vi "N4_X01.vi"(4 "error in":T15, 7 "Command":T16) -> (0 "error out":T15, 3 "Response":T13)   [LabVIEW 2018]
uses:
  MOKO_LabViewLibrary/MokoLowLevel/MokoLowLovelControl/MLLC_Command.ctl
  MOKO_LabViewLibrary/MokoLowLevel/MokoLowLovelControl/MLLC_Error.ctl
  MOKO_LabViewLibrary/MokoLowLevel/MokoLowLovelControl/MLLC_Mode.ctl
  MOKO_LabViewLibrary/MokoLowLevel/MokoLowLovelControl/MLLC_Response.ctl
  MOKO_LabViewLibrary/MokoLowLevel/MokoLowLovelControl/MLLC_DriverName.ctl
  MOKO_LabViewLibrary/MokoLowLevel/MokoLowLovelControl/MLLC_Request.ctl
  MOKO_LabViewLibrary/MokoLowLevel/MokoLowLovelControl/MLLC_ErrorCode.ctl
  MOKO_LabViewLibrary/MokoLowLevel/MokoLowLovelControl/MLLC_ResponseInit.ctl
  MOKO_LabViewLibrary/MokoLowLevel/MokoLowLovelControl/MLLC_ConnectCluster.ctl
  MOKO_LabViewLibrary/MokoLowLevel/MokoLowLovelControl/MLLC_InterfaceType.ctl
  MOKO_LabViewLibrary/MokoLowLevel/MokoLowLovelControl/MLLC_OpenedSession.ctl
  MOKO_LabViewLibrary/MokoLowLevel/MokoLowLovelControl/MLLC_InterfaceSettings.ctl
  MOKO_LabViewLibrary/MokoLowLevel/MokoLowLovelControl/MLLC_InterfaceKind.ctl
  MOKO_LabViewLibrary/MokoLowLevel/MokoLowLovelControl/MLLC_Boolean.ctl
  MOKO_LabViewLibrary/MokoLowLevel/MokoLowLovelControl/MLLC_Delay.ctl
panel:
  in  "Settings":T8={"Saved Data"=variant, "Permanent data"={"Connect"={"InterfaceType"=enum."VISA", "OpenedSession"="COM1", "InterfaceSettings"={"Interface"=enum."RS232", "EOS 4 read"=enum."LF (\\n)", "EOS 4 write"=enum."LF (\\n)", "TMO, ms"=10000, "Sett"=variant(cluster{"Baud Rate":u32, "Data Bits":u16, "Parity":u16, "Stop Bits":u16, "Flow Control":u16, "Eho":bool} {"Baud Rate"=75, "Data Bits"=0, "Parity"=0, "Stop Bits"=0, "Flow Control"=0, "Eho"=FALSE})}}, "RangeAuto"=TRUE, "SwitchOFF"=TRUE, "Range"=0.0}}
  in  "ResponseInit":T9="N4-101"
  in  "Error Code":T10=5470
  in  "Request":T11="IDN?"
  in  "Driver Name":T12="N4_101"
  in  "Mode":T14=enum."Check"
  # "Í4-X01"
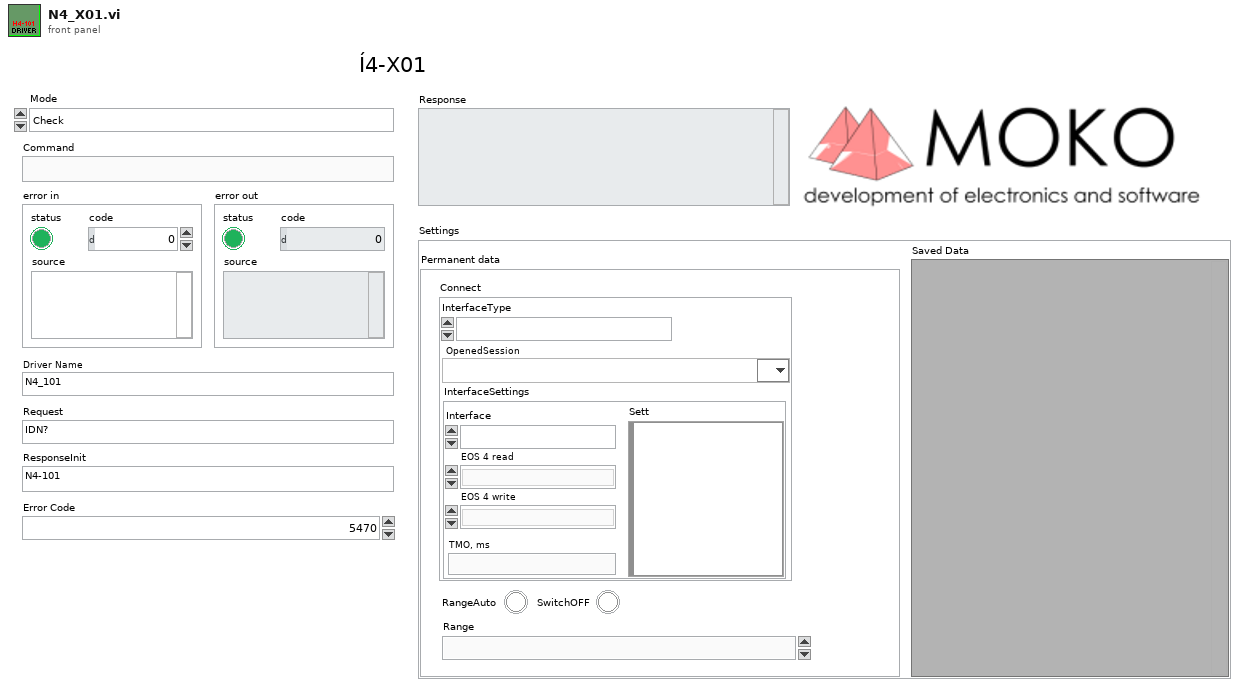
[diagram p1: front panel]
types:
  T1 = typedef "MLLC_ConnectCluster.ctl" = cluster{"InterfaceType":T2, "OpenedSession":T3, "InterfaceSettings":T4}
  T2 = typedef "MLLC_InterfaceType.ctl" = enum16{"VISA", "Prologix USB-GPIB"}
  T3 = typedef "MLLC_OpenedSession.ctl" = refnum<visa-resource-name>
  T4 = typedef "MLLC_InterfaceSettings.ctl" = cluster{"Interface":T5, "EOS 4 read":enum16{"Default (=EOS 4 write)", "CR (\\r)", "LF (\\n)", "None"}, "EOS 4 write":enum16{"CR+LF (\\r\\n)", "CR (\\r)", "LF (\\n)", "None"}, "TMO, ms":i32, "Sett":variant}
  T5 = typedef "MLLC_InterfaceKind.ctl" = enum16{"RS232", "GPIB", "USB", "Ethernet", "another"}
  T6 = typedef "MLLC_Boolean.ctl" = bool
  T7 = typedef "MLLC_Delay.ctl" = dbl
  T8 = cluster{"Saved Data":variant, "Permanent data":cluster{"Connect":T1, "RangeAuto":T6, "SwitchOFF":T6, "Range":T7}}
  T9 = typedef "MLLC_ResponseInit.ctl" = string
  T10 = typedef "MLLC_ErrorCode.ctl" = u32
  T11 = typedef "MLLC_Request.ctl" = string
  T12 = typedef "MLLC_DriverName.ctl" = string
  T13 = typedef "MLLC_Response.ctl" = string
  T14 = typedef "MLLC_Mode.ctl" = enum16{"get", "set", "close", "Init", "Check"}
  T15 = typedef "MLLC_Error.ctl" = errorcluster
  T16 = typedef "MLLC_Command.ctl" = string
  T17 = cluster{"Connect":T1, "RangeAuto":T6, "SwitchOFF":T6, "Range":T7}
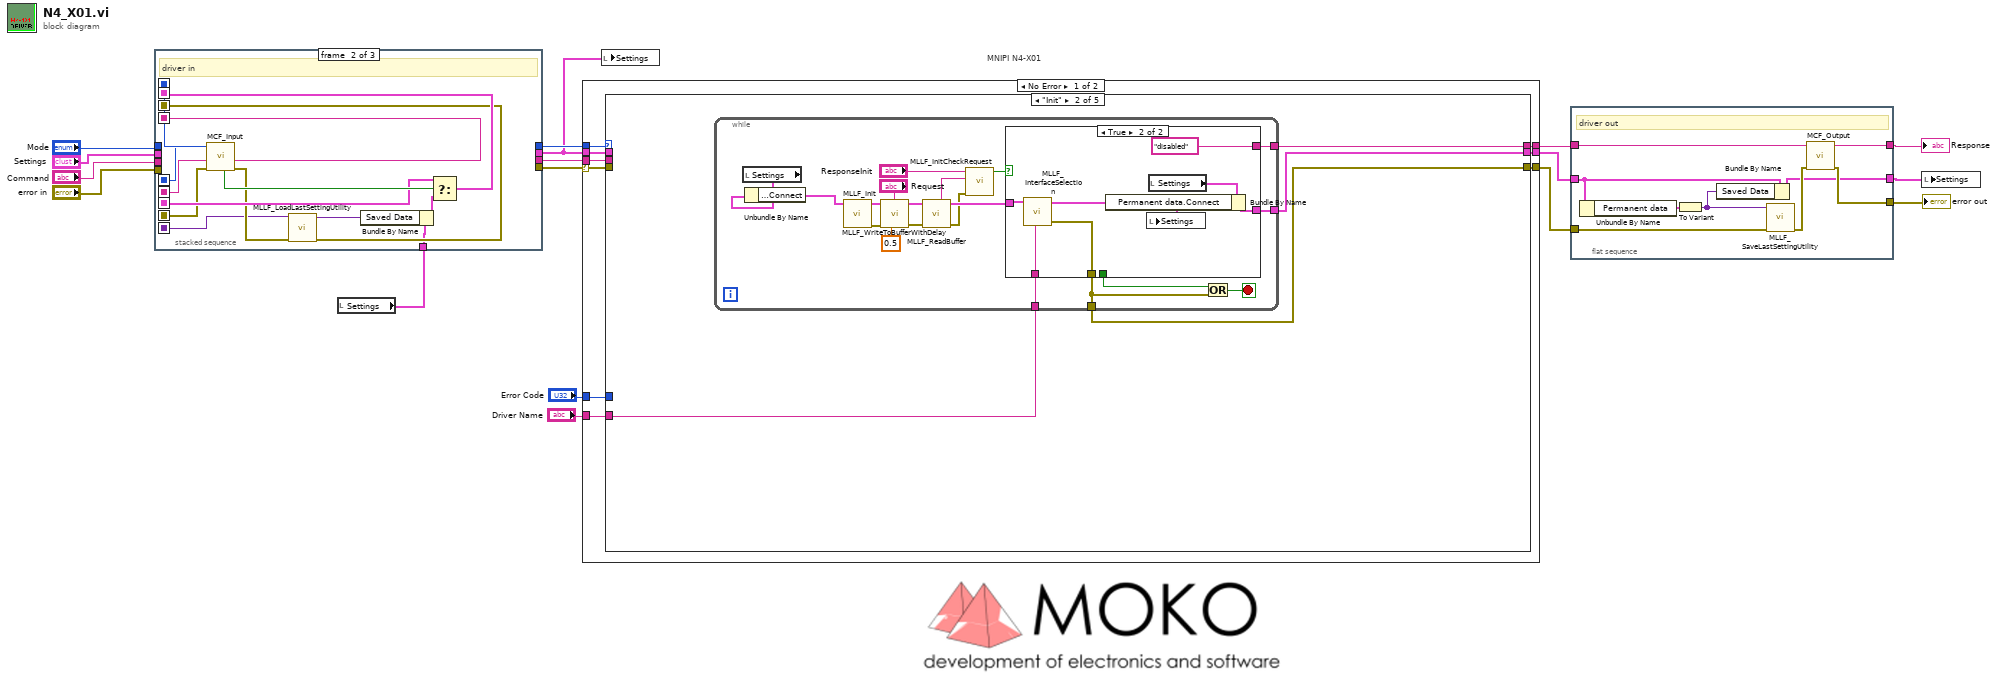
[diagram p0: block diagram]
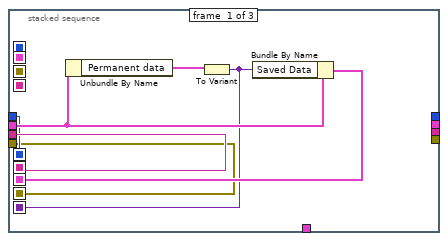
[diagram p2: hidden frame]
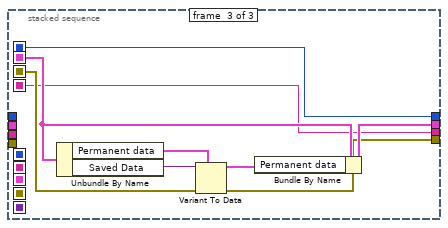
[diagram p3: hidden frame]
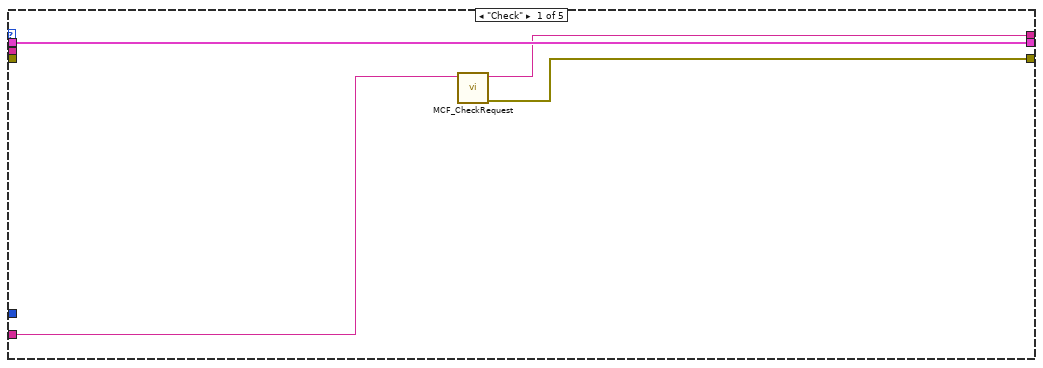
[diagram p4: hidden frame]
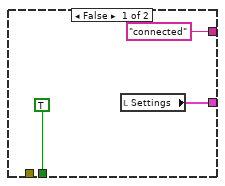
[diagram p5: hidden frame]
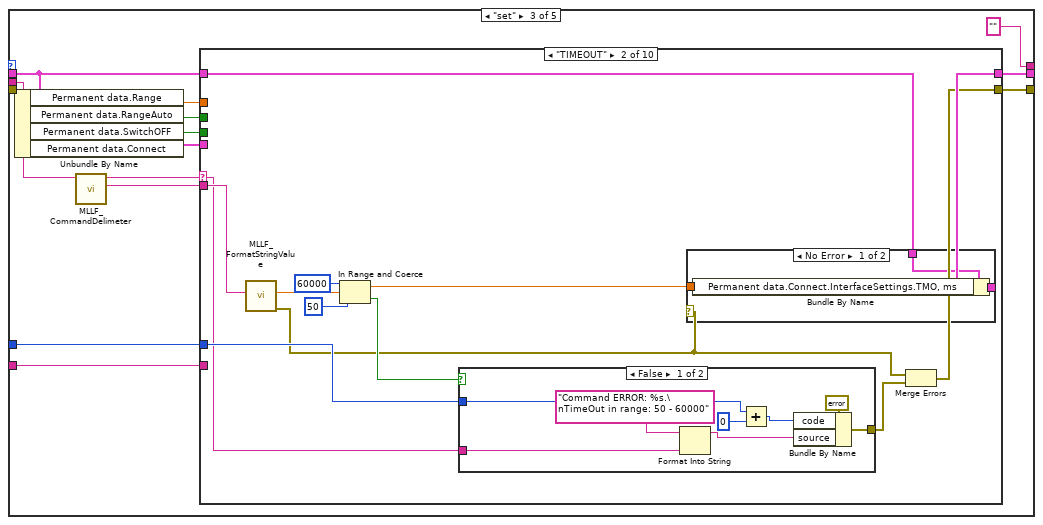
[diagram p6: hidden frame]
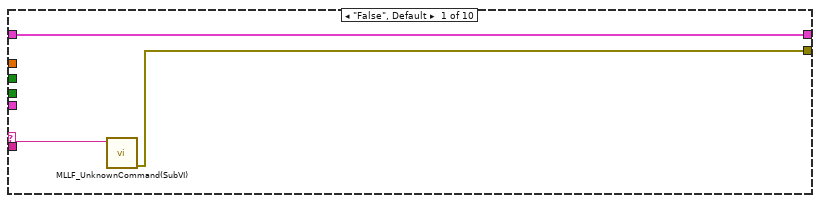
[diagram p7: hidden frame]
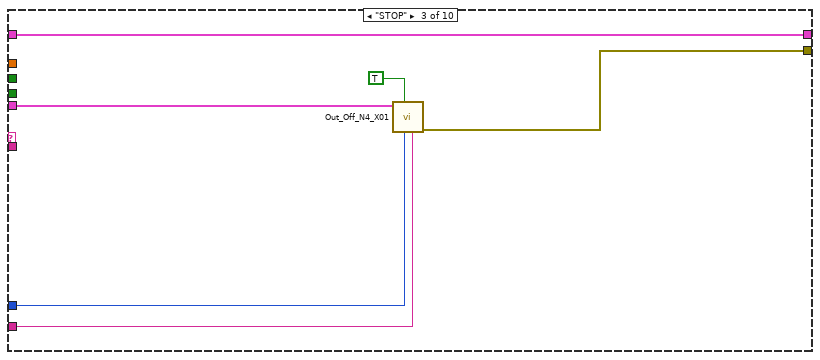
[diagram p10: hidden frame]
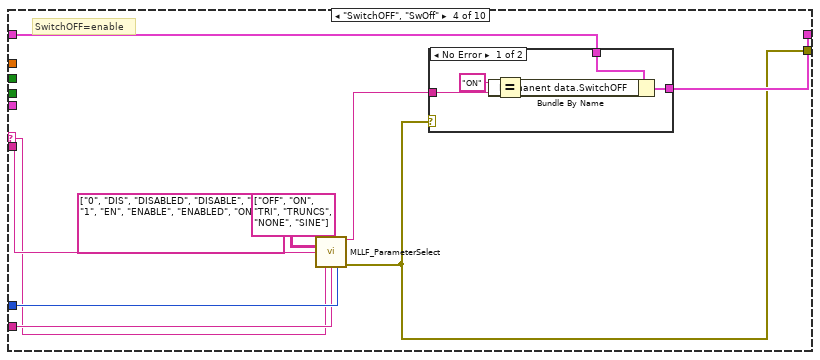
[diagram p11: hidden frame]
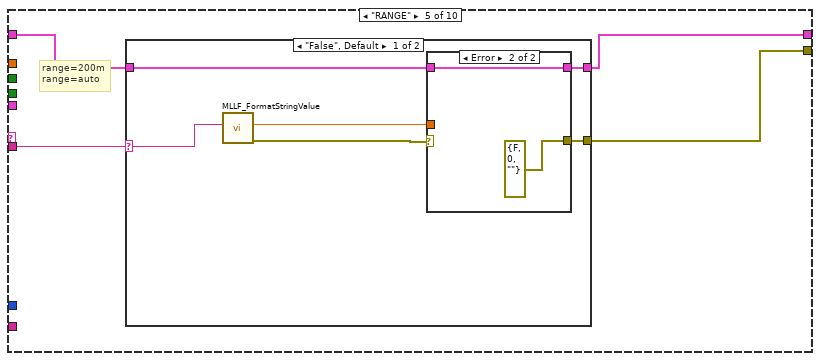
[diagram p13: hidden frame]
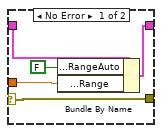
[diagram p14: hidden frame]
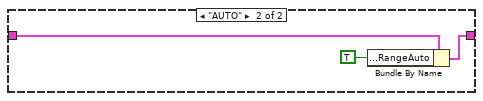
[diagram p15: hidden frame]
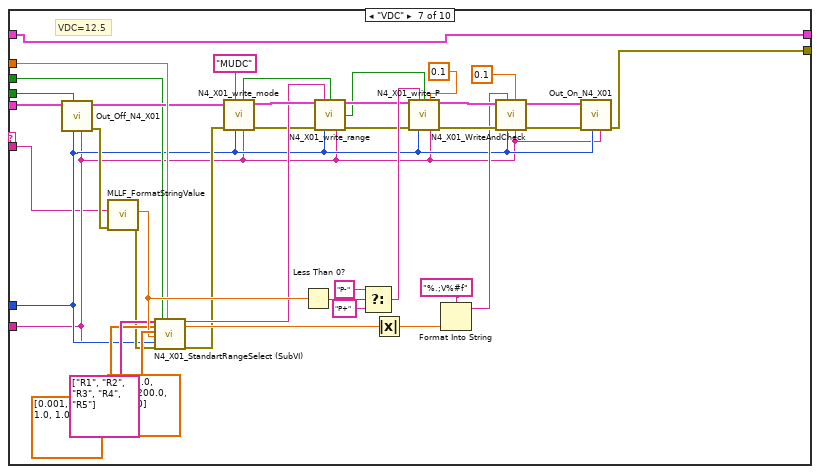
[diagram p17: hidden frame]
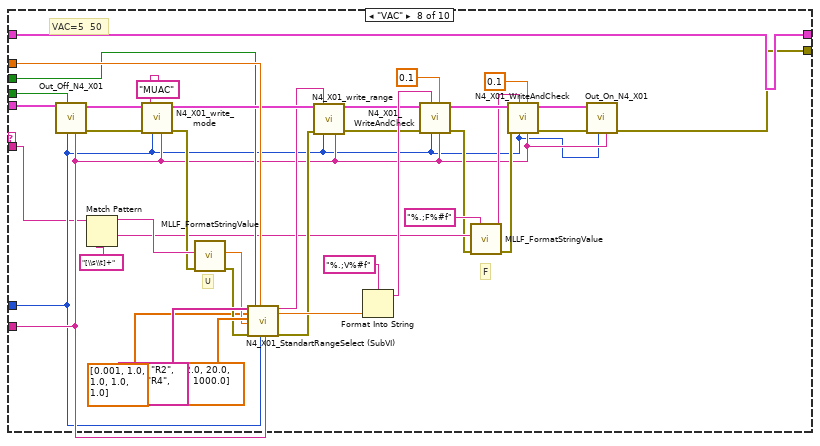
[diagram p18: hidden frame]
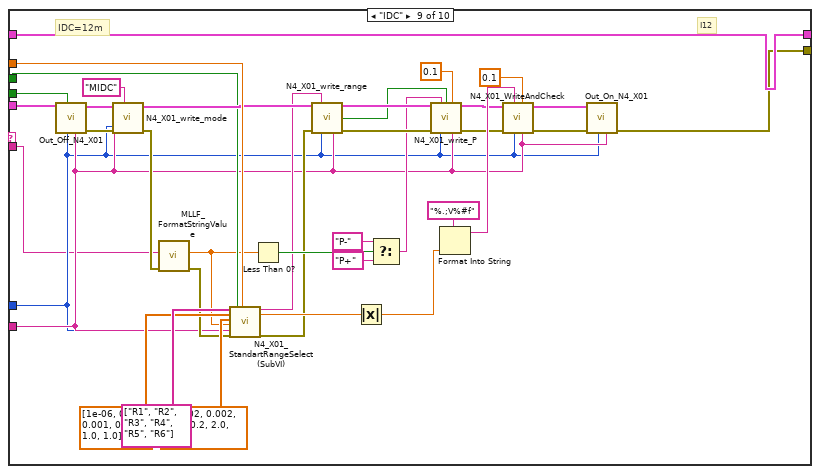
[diagram p19: hidden frame]
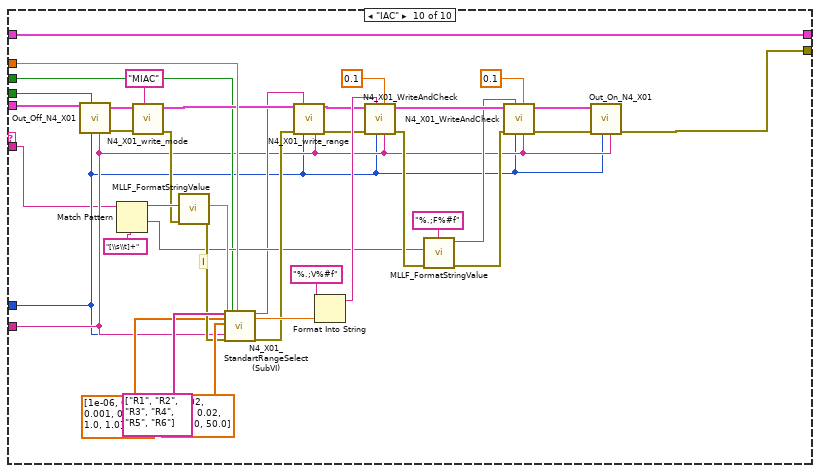
[diagram p20: hidden frame]
diagram:
  # "MNIPI N4-X01"
  n1 = local read "Settings"() -> (w7:T8)
  n2 = stacked-sequence {
    seq-local: [w20 _ _] -> [_ w36 _]
    seq-local: [w19 _ _] -> [_ w37 _]
    seq-local: [w22 _ _] -> [_ w32 _]
    seq-local: [w18 _ _] -> [_ w31 _]
    seq-local: [w21 _ _] -> [_ w27 _]
    seq-local: [_ w28 _] -> [_ _ w44]
    seq-local: [_ w38 _] -> [_ _ w41]
    seq-local: [_ w35 _] -> [_ _ w40]
    seq-local: [_ w34 _] -> [_ _ w45]
    tunnel: "Command" -> [w20 _ _]
    tunnel: "Mode" -> [w19 _ _]
    tunnel: "error in" -> [w18 _ _]
    tunnel: "Settings" -> [w23 _ _]
    tunnel: w7 -> [_ w26 _]
    tunnel: [_ _ w40] -> w9
    tunnel: [_ _ w43] -> w10
    tunnel: [_ _ w42] -> w8
    tunnel: [_ _ w41] -> w11
    frame #0 {
      n3 = Unbundle By Name(w23) -> ("Permanent data"=w24:T17)
      n4 = To Variant(anything=w24) -> (Variant=w21:variant)
      n5 = Bundle By Name(cluster=w23, "Saved Data"=w21) -> (w22:T8)
    }
    frame #1 {
      # "driver in"
      n6 = call "MCF_Input.vi"("Error In"=w31, "Command in"=w36, "Mode in"=w37) -> ("Error Out"=w30:errorcluster, "Command out"=w35:string, "Mode out"=w38:T14, "Boolean"=w33:bool)  [unwired: 5 in]
      n7 = call "MLLF_LoadLastSettingUtility.vi"("Error In"=w30, "Save data in"=w27) -> ("Error Out"=w28:errorcluster, "Save data out"=w25:variant)  [unwired: 8 in]
      n8 = Bundle By Name(cluster=w26, "Saved Data"=w25) -> (w29:T8)
      n9 = Select(t=w32, s=w33, f=w29) -> (s? t:f=w34:T8)
    }
    frame #2 {
      n10 = Unbundle By Name(w45) -> ("Permanent data"=w46:T17, "Saved Data"=w39:variant)
      n11 = Variant To Data(error in=w44, type=w46, Variant=w39) -> (data=w47:T17, error out=w42:errorcluster)
      n12 = Bundle By Name(cluster=w45, "Permanent data"=w47) -> (w43:T8)
    }
  }
  n13 = case shown="No Error" w8 {
    selector: w8 -> [w52 w369]
    tunnel: [w54 w369] -> w4
    tunnel: w11 -> [w56 _]
    tunnel: [w55 "" ("String")] -> w6
    tunnel: w9 -> [w53 _]
    tunnel: w10 -> [w49 w368]
    tunnel: "Error Code" -> [w51 _]
    tunnel: "Driver Name" -> [w50 _]
    tunnel: [w48 w368] -> w5
    frame No Error {
      n14 = case shown="\"Init\"" w56 {
        tunnel: [w58 w64 "" ("String") w332 "" ("String")] -> w55
        tunnel: [w59 w62 w96 w331 w365] -> w54
        tunnel: w53 -> [_ _ w106 w342 _]
        tunnel: w52 -> [_ _ _ _ _]
        tunnel: w51 -> [_ _ w105 w339 _]
        tunnel: w50 -> [w57 w61 w102 w338 _]
        tunnel: w49 -> [w60 _ w104 w341 w364]
        tunnel: [w60 w63 w103 w340 w364] -> w48
        frame "Check" {
          n15 = call "MCF_CheckRequest.vi"("Driver Name"=w57) -> ("Error Out"=w59:errorcluster, "Output String"=w58:string)  [unwired: 9 in]
        }
        frame "Init" {
          n16 = while {
            tunnel: [w76] -> w62
            tunnel: [w67] -> w63
            tunnel: [w66] -> w64
            tunnel: w61 -> [w65]
            stop <- w74 stop-if-true
            n17 = local read "Settings"() -> (w83:T8)
            n18 = Unbundle By Name(w83) -> ("Permanent data.Connect"=w77:T1)
            n19 = call "MLLF_Init.vi"("DriverConnect in"=w77) -> ("Error Out"=w79:errorcluster, "DriverConnect out"=w78:T1)  [unwired: 7 in]
            n20 = call "MLLF_WriteToBufferWithDelay.vi"("Delay Time ( 0,05 s)"=0.5 ("Delay Time (s)"), "Command"="Request", "Error In"=w79, "DriverConnect in"=w78) -> ("Error Out"=w72:errorcluster, "DriverConnect out"=w81:T1)  [unwired: 6 in]
            n21 = call "MLLF_ReadBuffer.vi"("Error In"=w72, "DriverConnect in"=w81) -> ("Error Out"=w69:errorcluster, "DriverConnect out"=w80:T1, "String"=w70:string)  [unwired: 6 in]
            n22 = call "MLLF_InitCheckRequest.vi"("error in (no error)"=w69, "Answer"=w70, "Response Init"="ResponseInit") -> ("Design"=w68:bool)  [unwired: 5 in, 3 out]
            n23 = case shown="True" w68 {
              tunnel: w80 -> [_ w92]
              tunnel: [_ w93] -> w76
              tunnel: [TRUE _] -> w75
              tunnel: [w84 w89] -> w67
              tunnel: ["connected" "disabled"] -> w66
              tunnel: w65 -> [_ w87]
              frame False {
                n24 = local read "Settings"() -> (w84:T8)
              }
              frame True {
                n25 = call "MLLF_InterfaceSelection.vi"("Driver Name"=w87, "DriverConnect in"=w92) -> ("error out"=w93:T15, "DriverConnect out"=w91:T1)  [unwired: 7 in, 1 out]
                n26 = local read "Settings"() -> (w90:T8)
                n27 = Bundle By Name(cluster=w90, "Permanent data.Connect"=w91) -> (w89:T8)
                n28 = local write "Settings"(w89) -> ()
              }
            }
            n29 = Or(x=w75, y=w76) -> (x .or. y?=w74:bool)
          }
        }
        frame "set" {
          n30 = Unbundle By Name(w104) -> ("Permanent data.Range"=w97:T7, "Permanent data.RangeAuto"=w98:T6, "Permanent data.SwitchOFF"=w99:T6, "Permanent data.Connect"=w100:T1)
          n31 = call "MLLF_CommandDelimeter.vi"("command with param"=w106) -> ("param 1"=w94:string, "command"=w95:string)  [unwired: 6 in, 3 out]
          n32 = case shown="\"TIMEOUT\"" w95 {
            selector: w95 -> [w108 w110 _ w141 _ _ _ _ _ _]
            tunnel: w94 -> [_ w113 _ w142 w160 _ w178 w218 w255 w294]
            tunnel: [w107 w116 w139 w145 w159 _ w179 w217 w256 w293] -> w96
            tunnel: w105 -> [_ w117 w137 w144 _ _ w182 w219 w258 w295]
            tunnel: w104 -> [w109 w121 w140 w147 w158 w177 w216 w253 w291 w329]
            tunnel: [w109 w122 w140 w146 w157 w177 w216 w253 w291 w329] -> w103
            tunnel: w100 -> [_ _ w136 _ _ _ w200 w254 w292 w330]
            tunnel: w102 -> [_ _ w138 w143 _ _ w181 w220 w259 w296]
            tunnel: w99 -> [_ _ _ _ _ _ w199 w245 w286 w320]
            tunnel: w98 -> [_ _ _ _ _ _ w193 w231 w266 w301]
            tunnel: w97 -> [_ _ _ _ _ _ w201 w237 w278 w312]
            frame "False", Default {
              n33 = call "MLLF_UnknownCommand(SubVI).vi"("Unknown command"=w108) -> ("error out"=w107:errorcluster)  [unwired: 10 in]
            }
            frame "TIMEOUT" {
              n34 = call "MLLF_FormatStringValue.vi"("String Value"=w113) -> ("error out"=w111:T15, "number"=w112:dbl)  [unwired: 8 in, 1 out]
              n35 = In Range and Coerce(upper limit=60000, x=w112, lower limit=50) -> (coerced(x)=w118:dbl, In Range?=w114:bool)
              n36 = case shown="False" w114 {
                tunnel: [w129 _] -> w115
                tunnel: w117 -> [w128 _]
                tunnel: w110 -> [w127 _]
                frame False {
                  n37 = Format Into String(format string="Command ERROR: %s.\nTimeOut in range: 50 - 60000", w127) -> (resulting string=w131:string)  [unwired: 2 in, 1 out]
                  n38 = Add(x=w128, y=0) -> (x+y=w132:T10)
                  n39 = Bundle By Name(cluster=errorcluster {"status"=TRUE, "code"=0, "source"=""} ("error out"), "code"=w132, "source"=w131) -> (w129:errorcluster)
                }
                frame True {
                }
              }
              n40 = case shown="No Error" w111 {
                tunnel: [w125 w126] -> w122
                tunnel: w121 -> [w124 w126]
                tunnel: w118 -> [w123 _]
                frame No Error {
                  n41 = Bundle By Name(cluster=w124, "Permanent data.Connect.InterfaceSettings.TMO, ms"=w123) -> (w125:T8)
                }
                frame Error {
                }
              }
              n42 = Merge Errors(w111, w115) -> (w116:errorcluster)
            }
            frame "STOP" {
              n43 = call "Out_Off_N4_X01.vi"("Driver Name"=w138, "Error Code"=w137, "SwitchOFF"=TRUE, "DriverConnect in"=w136) -> ("error out"=w139:T15)  [unwired: 6 in, 1 out]
            }
            frame "SwitchOFF", "SwOff" {
              # "SwitchOFF=enable"
              n44 = call "MLLF_ParameterSelect.vi"("Command to equipment"=string[] ["OFF", "ON", "TRI", "TRUNCS", "NONE", "SINE"] ("Parameters"), "Names"=string[][] [["0", "DIS", "DISABLED", "DISABLE", "OFF"], ["1", "EN", "ENABLE", "ENABLED", "ON"]], "Input"=w142, "Command"=w141, "Driver Name"=w143, "Error Code"=w144) -> ("Choice"=w150:string, "Error Out"=w145:errorcluster)  [unwired: 8 in]
              n45 = case shown="No Error" w145 {
                tunnel: w150 -> [w155 _]
                tunnel: w147 -> [w153 w156]
                tunnel: [w152 w156] -> w146
                frame No Error {
                  n46 = Equal?(x="ON", y=w155) -> (x = y?=w151:bool)
                  n47 = Bundle By Name(cluster=w153, "Permanent data.SwitchOFF"=w151) -> (w152:T8)
                }
                frame Error {
                }
              }
            }
            frame "RANGE" {
              # "range=200m\nrange=auto"
              n48 = case shown="\"False\", Default" w160 {
                selector: w160 -> [w166 _]
                tunnel: [w161 _] -> w159
                tunnel: [w164 w176] -> w157
                tunnel: w158 -> [w165 w175]
                frame "False", Default {
                  n49 = call "MLLF_FormatStringValue.vi"("String Value"=w166) -> ("error out"=w162:T15, "number"=w163:dbl)  [unwired: 8 in, 1 out]
                  n50 = case shown="Error" w162 {
                    selector: w162 -> [w167 _]
                    tunnel: w165 -> [w170 w173]
                    tunnel: [w169 w173] -> w164
                    tunnel: w163 -> [w168 _]
                    tunnel: [w167 errorcluster {"status"=FALSE, "code"=0, "source"=""} ("error IO")] -> w161
                    frame No Error {
                      n51 = Bundle By Name(cluster=w170, "Permanent data.RangeAuto"=FALSE ("RangeAuto"), "Permanent data.Range"=w168) -> (w169:T8)
                    }
                    frame Error {
                    }
                  }
                }
                frame "AUTO" {
                  n52 = Bundle By Name(cluster=w175, "Permanent data.RangeAuto"=TRUE ("RangeAuto")) -> (w176:T8)
                }
              }
            }
            frame "<----MAIN FUNCTIONS---->" {
            }
            frame "VDC" {
              # "VDC=12.5"
              n53 = call "Out_Off_N4_X01.vi"("Driver Name"=w181, "Error Code"=w182, "SwitchOFF"=w199, "DriverConnect in"=w200) -> ("error out"=w189:T15, "DriverConnect out"=w195:T1)  [unwired: 6 in]
              n54 = call "MLLF_FormatStringValue.vi"("error in"=w189, "String Value"=w178) -> ("error out"=w191:T15, "number"=w214:dbl)  [unwired: 7 in, 1 out]
              n55 = call "N4_X01_StandartRangeSelect (SubVI).vi"("Range Command"=string[] ["R1", "R2", "R3", "R4", "R5"] ("RangeCommand"), "Scale Array"=dbl[] [0.001, 1.0, 1.0, 1.0, 1.0] ("ScaleArray"), "Range Digit"=dbl[] [0.2, 2.0, 20.0, 200.0, 1000.0] ("RangeDigit"), "Control Point"=w214, "Error In"=w191, "RangeAuto"=w193, "Range"=w201, "Error Code"=w182, "Driver Name"=w181) -> ("Range Out"=w194:string, "Scaled value"=w212:dbl, "Error Out"=w188:errorcluster)  [unwired: 8 in]
              n56 = call "N4_X01_write_mode.vi"("Driver Name"=w181, "Error Code"=w182, "Command"="MUDC" ("String"), "error in"=w188, "DriverConnect in"=w195) -> ("error out"=w187:T15, "DriverConnect out"=w198:T1, "ModeWasChacged"=w186:T6)  [unwired: 4 in]
              n57 = Less Than 0?(x=w214) -> (x < 0?=w211:bool)
              n58 = call "N4_X01_write_range.vi"("DriverConnect in"=w198, "Command range"=w194, "ModeIsChanged?"=w186, "error in"=w187, "Error Code"=w182, "Driver Name"=w181) -> ("DriverConnect out"=w197:T1, "RangeWasChanged"=w190:T6, "error out"=w196:T15)  [unwired: 7 in]
              n59 = Select(t="P-" ("String"), s=w211, f="P+" ("String")) -> (s? t:f=w208:string)
              n60 = Absolute Value(x=w212) -> (abs(x)=w205:dbl)
              n61 = call "N4_X01_write_P.vi"("DriverConnect in"=w197, "P"=w208, "RangeIsChanged?"=w190, "Command Time (s)"=0.1, "error in"=w196, "Error Code"=w182, "Driver Name"=w181) -> ("DriverConnect out"=w206:T1, "error out"=w207:T15)  [unwired: 7 in]
              n62 = Format Into String(format string="%.;V%#f", w205) -> (resulting string=w203:string)  [unwired: 2 in, 1 out]
              n63 = call "N4_X01_WriteAndCheck.vi"("Driver Name"=w181, "Command Time (s)"=0.1, "Error Code"=w182, "Command"=w203, "error in"=w207, "DriverConnect in"=w206) -> ("error out"=w183:T15, "DriverConnect out"=w184:T1)  [unwired: 4 in]
              n64 = call "Out_On_N4_X01.vi"("Driver Name"=w181, "Error Code"=w182, "error in"=w183, "DriverConnect in"=w184) -> ("error out"=w179:T15)  [unwired: 6 in, 1 out]
            }
            frame "VAC" {
              # "VAC=5  50"
              # "F"
              # "U"
              n65 = call "Out_Off_N4_X01.vi"("Driver Name"=w220, "Error Code"=w219, "SwitchOFF"=w245, "DriverConnect in"=w254) -> ("error out"=w230:T15, "DriverConnect out"=w236:T1)  [unwired: 6 in]
              n66 = Match Pattern(string=w218, regular expression="[\\s\\t]+") -> (before substring=w238:string, after substring=w227:string)  [unwired: 1 in, 2 out]
              n67 = call "N4_X01_write_mode.vi"("Driver Name"=w220, "Error Code"=w219, "Command"="MUAC" ("String"), "error in"=w230, "DriverConnect in"=w236) -> ("error out"=w229:T15, "DriverConnect out"=w235:T1)  [unwired: 4 in, 1 out]
              n68 = call "MLLF_FormatStringValue.vi"("error in"=w229, "String Value"=w238) -> ("error out"=w247:T15, "number"=w248:dbl)  [unwired: 7 in, 1 out]
              n69 = call "N4_X01_StandartRangeSelect (SubVI).vi"("Range Command"=string[] ["R1", "R2", "R3", "R4", "R5"] ("RangeCommand"), "Scale Array"=dbl[] [0.001, 1.0, 1.0, 1.0, 1.0] ("ScaleArray"), "Range Digit"=dbl[] [0.2, 2.0, 20.0, 200.0, 1000.0] ("RangeDigit"), "Control Point"=w248, "Error In"=w247, "RangeAuto"=w231, "Range"=w237, "Error Code"=w219, "Driver Name"=w220) -> ("Range Out"=w234:string, "Scaled value"=w242:dbl, "Error Out"=w228:errorcluster)  [unwired: 8 in]
              n70 = call "N4_X01_write_range.vi"("DriverConnect in"=w235, "Command range"=w234, "error in"=w228, "Error Code"=w219, "Driver Name"=w220) -> ("DriverConnect out"=w233:T1, "error out"=w232:T15)  [unwired: 8 in, 1 out]
              n71 = Format Into String(format string="%.;V%#f", w242) -> (resulting string=w239:string)  [unwired: 2 in, 1 out]
              n72 = call "N4_X01_WriteAndCheck.vi"("Driver Name"=w220, "Command Time (s)"=0.1, "Error Code"=w219, "Command"=w239, "error in"=w232, "DriverConnect in"=w233) -> ("error out"=w226:T15, "DriverConnect out"=w244:T1)  [unwired: 4 in]
              n73 = call "MLLF_FormatStringValue.vi"("error in"=w226, "String Value"=w227, "Format"="%.;F%#f" ("format string")) -> ("error out"=w243:T15, "String Value Formated"=w240:T16)  [unwired: 6 in, 1 out]
              n74 = call "N4_X01_WriteAndCheck.vi"("Driver Name"=w220, "Command Time (s)"=0.1, "Error Code"=w219, "Command"=w240, "error in"=w243, "DriverConnect in"=w244) -> ("error out"=w221:T15, "DriverConnect out"=w222:T1)  [unwired: 4 in]
              n75 = call "Out_On_N4_X01.vi"("Driver Name"=w220, "Error Code"=w219, "error in"=w221, "DriverConnect in"=w222) -> ("error out"=w217:T15)  [unwired: 6 in, 1 out]
            }
            frame "IDC" {
              # "IDC=12m"
              # "I12"
              n76 = call "Out_Off_N4_X01.vi"("Driver Name"=w259, "Error Code"=w258, "SwitchOFF"=w286, "DriverConnect in"=w292) -> ("error out"=w270:T15, "DriverConnect out"=w272:T1)  [unwired: 6 in]
              n77 = call "N4_X01_write_mode.vi"("Driver Name"=w259, "Error Code"=w258, "Command"="MIDC" ("String"), "error in"=w270, "DriverConnect in"=w272) -> ("error out"=w269:T15, "DriverConnect out"=w275:T1)  [unwired: 4 in, 1 out]
              n78 = call "MLLF_FormatStringValue.vi"("error in"=w269, "String Value"=w255) -> ("error out"=w285:T15, "number"=w263:dbl)  [unwired: 7 in, 1 out]
              n79 = call "N4_X01_StandartRangeSelect (SubVI).vi"("Range Command"=string[] ["R1", "R2", "R3", "R4", "R5", "R6"] ("RangeCommand"), "Scale Array"=dbl[] [1e-06, 0.001, 0.001, 0.001, 1.0, 1.0] ("ScaleArray"), "Range Digit"=dbl[] [0.0002, 0.002, 0.02, 0.2, 2.0, 50.0] ("RangeDigit"), "Control Point"=w263, "Error In"=w285, "RangeAuto"=w266, "Range"=w278, "Error Code"=w258, "Driver Name"=w259) -> ("Range Out"=w271:string, "Scaled value"=w287:dbl, "Error Out"=w268:errorcluster)  [unwired: 8 in]
              n80 = Less Than 0?(x=w263) -> (x < 0?=w282:bool)
              n81 = call "N4_X01_write_range.vi"("DriverConnect in"=w275, "Command range"=w271, "error in"=w268, "Error Code"=w258, "Driver Name"=w259) -> ("DriverConnect out"=w276:T1, "RangeWasChanged"=w264:T6, "error out"=w277:T15)  [unwired: 8 in]
              n82 = Absolute Value(x=w287) -> (abs(x)=w279:dbl)
              n83 = Select(t="P-" ("String"), s=w282, f="P+" ("String")) -> (s? t:f=w267:string)
              n84 = call "N4_X01_write_P.vi"("DriverConnect in"=w276, "P"=w267, "RangeIsChanged?"=w264, "Command Time (s)"=0.1, "error in"=w277, "Error Code"=w258, "Driver Name"=w259) -> ("DriverConnect out"=w274:T1, "error out"=w273:T15)  [unwired: 7 in]
              n85 = Format Into String(format string="%.;V%#f", w279) -> (resulting string=w281:string)  [unwired: 2 in, 1 out]
              n86 = call "N4_X01_WriteAndCheck.vi"("Driver Name"=w259, "Command Time (s)"=0.1, "Error Code"=w258, "Command"=w281, "error in"=w273, "DriverConnect in"=w274) -> ("error out"=w260:T15, "DriverConnect out"=w261:T1)  [unwired: 4 in]
              n87 = call "Out_On_N4_X01.vi"("Driver Name"=w259, "Error Code"=w258, "error in"=w260, "DriverConnect in"=w261) -> ("error out"=w256:T15)  [unwired: 6 in, 1 out]
            }
            frame "IAC" {
              # "I"
              n88 = call "Out_Off_N4_X01.vi"("Driver Name"=w296, "Error Code"=w295, "SwitchOFF"=w320, "DriverConnect in"=w330) -> ("error out"=w306:T15, "DriverConnect out"=w308:T1)  [unwired: 6 in]
              n89 = Match Pattern(string=w294, regular expression="[\\s\\t]+") -> (before substring=w327:string, after substring=w303:string)  [unwired: 1 in, 2 out]
              n90 = call "N4_X01_write_mode.vi"("Command"="MIAC" ("String"), "error in"=w306, "DriverConnect in"=w308) -> ("error out"=w305:T15, "DriverConnect out"=w311:T1)  [unwired: 6 in, 1 out]
              n91 = call "MLLF_FormatStringValue.vi"("error in"=w305, "String Value"=w327) -> ("error out"=w323:T15, "number"=w322:dbl)  [unwired: 7 in, 1 out]
              n92 = call "N4_X01_StandartRangeSelect (SubVI).vi"("Range Command"=string[] ["R1", "R2", "R3", "R4", "R5", "R6"] ("RangeCommand"), "Scale Array"=dbl[] [1e-06, 0.001, 0.001, 0.001, 1.0, 1.0] ("ScaleArray"), "Range Digit"=dbl[] [0.0002, 0.002, 0.02, 0.2, 2.0, 50.0] ("RangeDigit"), "Control Point"=w322, "Error In"=w323, "RangeAuto"=w301, "Range"=w312, "Error Code"=w295, "Driver Name"=w296) -> ("Range Out"=w302:string, "Scaled value"=w315:dbl, "Error Out"=w304:errorcluster)  [unwired: 8 in]
              n93 = call "N4_X01_write_range.vi"("DriverConnect in"=w311, "Command range"=w302, "error in"=w304, "Error Code"=w295, "Driver Name"=w296) -> ("DriverConnect out"=w310:T1, "error out"=w309:T15)  [unwired: 8 in, 1 out]
              n94 = Format Into String(format string="%.;V%#f", w315) -> (resulting string=w319:string)  [unwired: 2 in, 1 out]
              n95 = call "N4_X01_WriteAndCheck.vi"("Driver Name"=w296, "Command Time (s)"=0.1, "Error Code"=w295, "Command"=w319, "error in"=w309, "DriverConnect in"=w310) -> ("error out"=w314:T15, "DriverConnect out"=w318:T1)  [unwired: 4 in]
              n96 = call "MLLF_FormatStringValue.vi"("error in"=w314, "String Value"=w303, "Format"="%.;F%#f" ("format string")) -> ("error out"=w313:T15, "String Value Formated"=w317:T16)  [unwired: 6 in, 1 out]
              n97 = call "N4_X01_WriteAndCheck.vi"("Driver Name"=w296, "Command Time (s)"=0.1, "Error Code"=w295, "Command"=w317, "error in"=w313, "DriverConnect in"=w318) -> ("error out"=w297:T15, "DriverConnect out"=w298:T1)  [unwired: 4 in]
              n98 = call "Out_On_N4_X01.vi"("Driver Name"=w296, "Error Code"=w295, "error in"=w297, "DriverConnect in"=w298) -> ("error out"=w293:T15)  [unwired: 6 in, 1 out]
            }
          }
        }
        frame "get" {
          n99 = Unbundle By Name(w341) -> ("Permanent data.Connect"=w335:T1)
          n100 = call "MLLF_CommandDelimeter.vi"("command with param"=w342) -> ("param 1"=w333:string, "command"=w334:string)  [unwired: 6 in, 3 out]
          n101 = case shown="\"AMPL\", \"AMPLITUDE\"" w334 {
            selector: w334 -> [w344 _ _]
            tunnel: w333 -> [_ _ _]
            tunnel: [w343 _ w351] -> w337
            tunnel: w339 -> [_ _ _]
            tunnel: [w347 w350 w362] -> w340
            tunnel: w341 -> [w347 w350 w362]
            tunnel: [w345 w348 w361] -> w336
            tunnel: w335 -> [_ _ w354]
            tunnel: w338 -> [_ _ _]
            frame "False", Default {
              n102 = call "MLLF_UnknownCommand(SubVI).vi"("Unknown command"=w344) -> ("error out"=w343:errorcluster)  [unwired: 10 in]
              n103 = Build Array(0 ("TimeOut")) -> (w345:i32[])
            }
            frame "TIMEOUT" {
              n104 = Unbundle By Name(w350) -> ("Permanent data.Connect.InterfaceSettings.TMO, ms"=w349:i32)
              n105 = Build Array(w349) -> (w348:i32[])
            }
            frame "AMPL", "AMPLITUDE" {
              n106 = call "MLLF_WriteToBuffer.vi"("String"="V?" ("Error Query"), "DriverConnect in"=w354) -> ("error out"=w359:T15, "DriverConnect out"=w355:T1)  [unwired: 6 in]
              n107 = call "500ms12"("error in (no error)"=w359) -> ("error out"=w360:errorcluster)  [unwired: 10 in]
              n108 = call "MLLF_ReadBuffer.vi"("Error In"=w360, "DriverConnect in"=w355) -> ("Error Out"=w352:errorcluster, "String"=w357:string)  [unwired: 6 in, 1 out]
              n109 = call "MLLF_FormatStringValue.vi"("error in"=w352, "String Value"=w357, "Format"="%#e" ("format string")) -> ("error out"=w351:T15, "number"=w353:dbl)  [unwired: 6 in, 1 out]
              n110 = Build Array(w353) -> (w361:dbl[])
            }
          }
          n111 = call "MLLF_FormatOutputValueWithUnits.vi"("error in"=w337, "ValuesIn"=w336) -> ("error out"=w331:T15, "Result string"=w332:T16)  [unwired: 8 in]
        }
        frame "close" {
          n112 = Unbundle By Name(w364) -> ("Permanent data.Connect.OpenedSession"=w366:T3)
          n113 = VISA Close(VISA resource name=w366) -> (error out=w365:errorcluster)  [unwired: 1 in]
        }
      }
    }
    frame Error {
    }
  }
  n114 = local write "Settings"(w10) -> ()
  n115 = flat-sequence {
    tunnel: [w378] -> w1
    tunnel: [w377] -> w3
    tunnel: w6 -> [w376]
    tunnel: w4 -> [w375]
    tunnel: w5 -> [w371]
    tunnel: [w373] -> w2
    frame #0 {
      # "driver out"
      n116 = Unbundle By Name(w371) -> ("Permanent data"=w370:T17)
      n117 = To Variant(anything=w370) -> (Variant=w372:variant)
      n118 = Bundle By Name(cluster=w371, "Saved Data"=w372) -> (w373:T8)
      n119 = call "MLLF_SaveLastSettingUtility.vi"("error in"=w375, "Saved Data"=w372) -> ("error out"=w374:T15)  [unwired: 8 in, 1 out]
      n120 = call "MCF_Output.vi"("Error In"=w374, "Input"=w376) -> ("Error Out"=w377:errorcluster, "Output"=w378:string)  [unwired: 8 in]
    }
  }
  n121 = local write "Settings"(w2) -> ()
  "error out" <- w3
  "Response" <- w1
